vi "Grab with Bayer Decoding -ajg.vi"() -> ()   [LabVIEW 2020]
doc: "The Grab with Bayer Decoding VI acquires images continuously and displays the decoded Bayer image as an RGB image in an image control on the front panel. \n\nIMAQ Create Bayer LUT configures the gains to apply to the color planes. Refer to the Bayer decoding documentation in the White Balancing Utility for more information about setting the appropriate gains. Initialize the LUT only once to minimize decoding time. IMAQ Bayer Color Decode decodes a monochrome image to create the RGB image. An image control displays the RGB image on the front panel. After exiting the loop, IMAQ Extract Buffer releases the last extracted buffer. IMAQ Close releases resources associated with the acquisition, and IMAQ Dispose frees the buffers used for acquisition and Bayer decoding."
panel:
  out "error out 4":errorcluster
  out "error out 3":errorcluster
  out "error out 2":errorcluster
  out "Image 2":T1(plugin-control)
  out "error out":errorcluster
  in  "milliseconds to wait":u32=200
  in  "File Path":path=path "c:/temp"
  in  "Save":bool
  in  "Bayer Decoding Parameters":T2={"Bayer Pattern"=0, "Decode Method"=0, "Red Gain"=1.0, "Blue Gain"=1.0, "Green Gain"=1.0} {"Green Gain" min=0.0 max=3.99 step=0.01; "Blue Gain" min=0.0 max=3.99 step=0.01; "Red Gain" min=0.0 max=3.99 step=0.01; "Decode Method" items=["Bilinear", "VNG"]; "Bayer Pattern" items=["GBGB::RGRG", "GRGR::BGBG", "BGBG::GRGR", "RGRG::GBGB"]}
  out "Image":T1(plugin-control)
  out "Buffer Number":u32
  in  "Interface Name":string="img0"
  in  "Stop":bool
  # "Overview: Demonstrates how to perform a continuous acquisition and decode Bayer images to a color image.\nRequirements: Vision Acquisition Software, IMAQ frame grabber.\nInstructions: \n1. Select the IMAQ frame grabber Interface Name.\n2. Run the VI.\n3. If the camera file associated with the Interface Name does not already have Bayer settings defined, you can adjust the gains and Bayer Pattern. Otherwise, you can only adjust the gains."
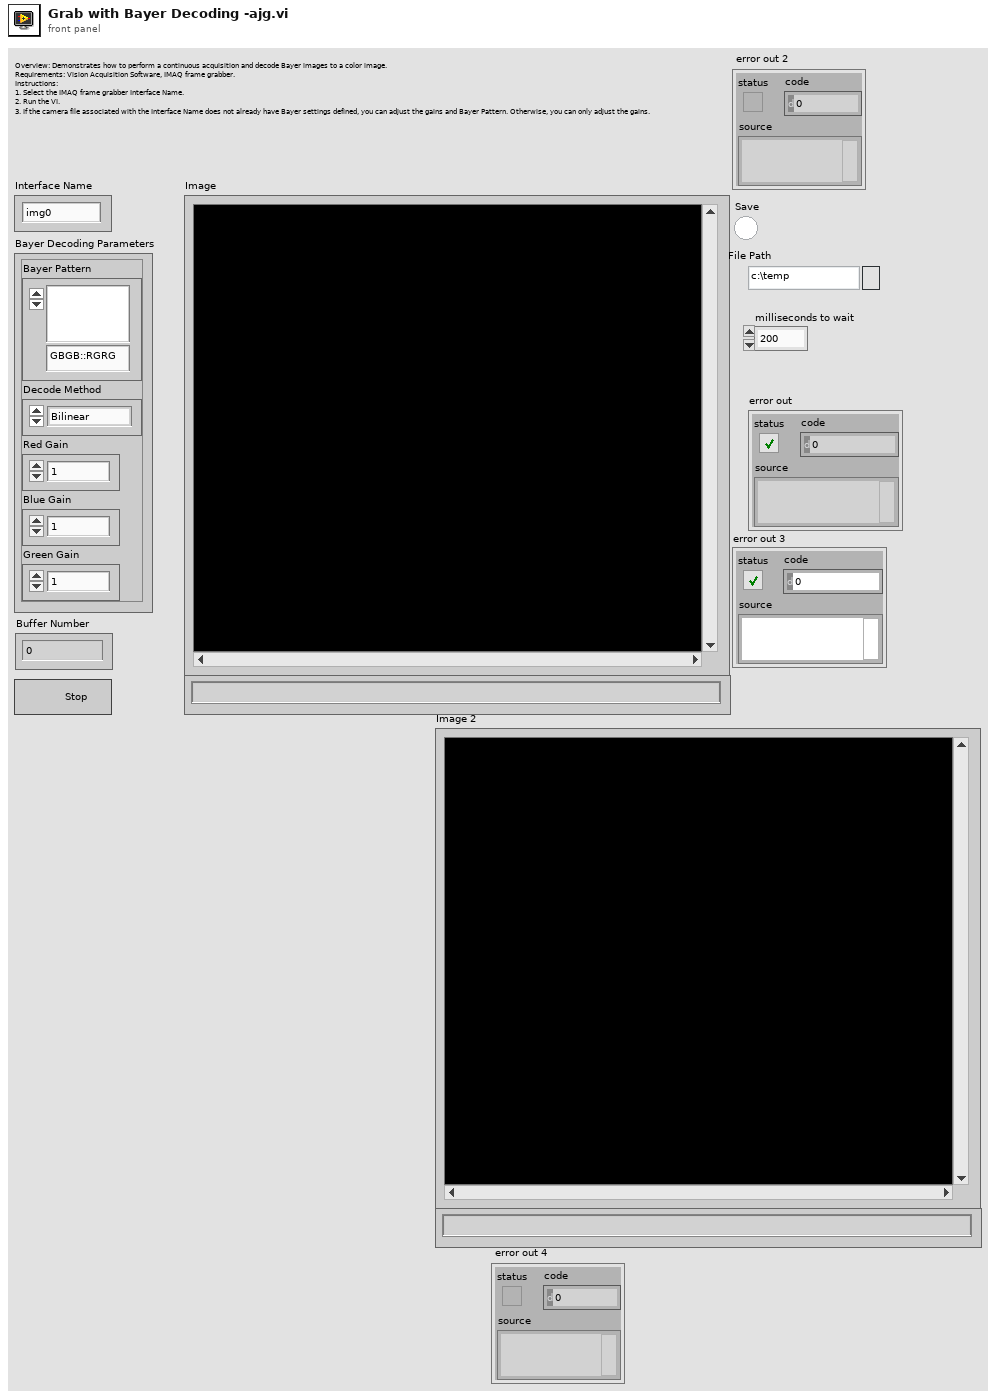
[diagram p1: front panel]
types:
  T1 = typedef "IMAQ Image.ctl" = refnum<image>
  T2 = cluster{"Bayer Pattern":i32, "Decode Method":i32, "Red Gain":dbl, "Blue Gain":dbl, "Green Gain":dbl}
  T3 = typedef "Image Type" = u32
  T4 = enum8{"Enabled", "Disabled", "Disabled and Grayed Out"}
  T5 = cluster{"Bayer Pattern":i32, "Decode Method":i32, "Bayer Red Gain":dbl, "Bayer Green Gain":dbl, "Bayer Blue Gain":dbl}
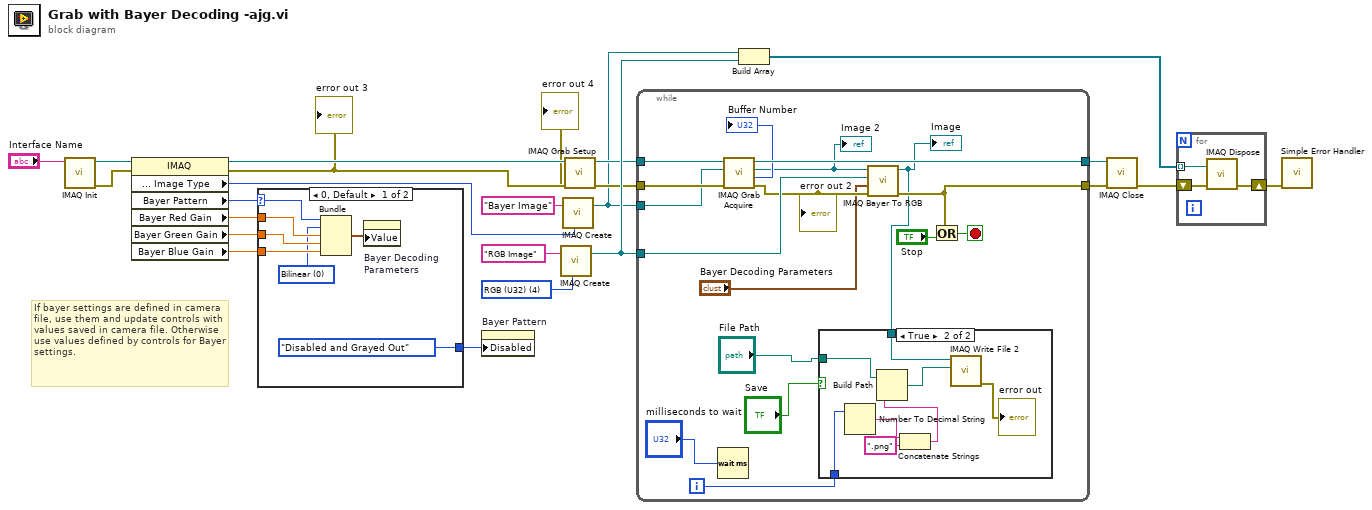
[diagram p0: block diagram]
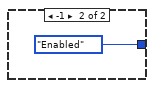
[diagram p2: hidden frame]
diagram:
  w18 = T3 4 items=["Grayscale (U8)", "Grayscale (I16)", "Grayscale (SGL)", "Complex (CSG)", "RGB (U32)", "HSL (U32)", "RGB (U64)", "Grayscale (U16)"] ("Image Type")
  # "If bayer settings are defined in camera file, use them and update controls with values saved in camera file. Otherwise use values defined by controls for Bayer settings."
  n1 = call <vilib>:"IMAQ Init.vi"("Interface Name"="Interface Name") -> ("error out"=w11:errorcluster, "IMAQ Session Out"=w12:refnum<k11>)  [unwired: 1 in, 8 out]
  n2 = property class="IMAQ"(reference=w12, error in=w11) -> (reference out=w10:refnum<k11>, error out=w9:errorcluster, "Image Parameters : Image Type"=w5:u32, "Bayer Pattern"=w16:i32, "Bayer Red Gain"=w15:dbl, "Bayer Green Gain"=w14:dbl, "Bayer Blue Gain"=w13:dbl)
  "error out 3" <- w9
  n3 = case shown="0, Default" w16 {
    selector: w16 -> [w26 _]
    tunnel: w15 -> [w29 _]
    tunnel: w14 -> [w28 _]
    tunnel: w13 -> [w27 _]
    tunnel: [T4."Disabled and Grayed Out" ("Disabled") T4."Enabled" ("Disabled")] -> w4
    frame 0, Default {
      w24 = 0 items=["Bilinear", "VNG"] ("Decode Method")
      n4 = Bundle("Bayer Pattern"=w26, "Decode Method"=w24, "Bayer Red Gain"=w29, "Bayer Green Gain"=w28, "Bayer Blue Gain"=w27) -> (w25:T5)  [unwired: 1 in]
      n5 = property on="Bayer Decoding Parameters" class="Clust (strict)"("Value"=w25) -> ()  [unwired: 2 in, 2 out]
    }
    frame -1 {
    }
  }
  n6 = property on="Bayer Pattern" class="Ring (strict)"("Disabled"=w4) -> ()  [unwired: 2 in, 2 out]
  n7 = call "IMAQ Create"("Image Name"="RGB Image", "Image Type"=w18) -> ("New Image"=w17:T1)  [unwired: 2 in, 2 out]
  n8 = call "IMAQ Create"("Image Name"="Bayer Image", "Image Type"=w5) -> ("New Image"=w3:T1)  [unwired: 2 in, 2 out]
  n9 = call <vilib>:"IMAQ Grab Setup.vi"("error in (no error)"=w9, "IMAQ Session In"=w10) -> ("error out"=w8:errorcluster, "IMAQ Session Out"=w7:refnum<k11>)  [unwired: 8 in]
  "error out 4" <- w8
  n10 = while {
    tunnel: w17 -> [w41]
    tunnel: [w45] -> w2
    tunnel: w7 -> [w46]
    tunnel: w8 -> [w44]
    tunnel: [w40] -> w1
    tunnel: w3 -> [w42]
    i -> [w35]
    stop <- w47 stop-if-true
    n11 = Wait (ms)(milliseconds to wait="milliseconds to wait") -> ()  [unwired: 1 out]
    n12 = call <vilib>:"IMAQ Grab Acquire.vi"("error in (no error)"=w44, "Image In"=w42, "IMAQ Session In"=w46) -> ("error out"=w39:errorcluster, "Acquired Buffer Number"=→"Buffer Number":u32, "Image Out"=w32:T1, "IMAQ Session Out"=w45:refnum<k11>)  [unwired: 5 in]
    "Image 2" <- w32
    "error out 2" <- w39
    n13 = call "IMAQ Bayer To RGB"("error in (no error)"=w39, "Bayer Parameters"="Bayer Decoding Parameters", "Image Dst"=w41, "Image Src"=w32) -> ("error out"=w40:errorcluster, "Image Dst Out"=w33:T1)  [unwired: 6 in]
    "Image" <- w33
    n14 = case shown="True" "Save" {
      tunnel: "File Path" -> [_ w56]
      tunnel: w35 -> [_ w53]
      tunnel: w33 -> [_ w51]
      frame False {
      }
      frame True {
        n15 = Number To Decimal String(number=w53) -> (decimal integer string=w55:string)  [unwired: 1 in]
        n16 = Concatenate Strings(w55, ".png" ("string")) -> (w52:string)
        n17 = Build Path(base path=w56, name or relative path=w52) -> (appended path=w50:path)
        n18 = call-poly "IMAQ Write File 2"("File Path"=w50, "Image"=w51) -> ("error out"=→"error out":errorcluster)  [unwired: 8 in, 1 out]
      }
    }
    n19 = Or(x=w40, y="Stop") -> (x .or. y?=w47:bool)
  }
  n20 = Build Array(w3, w17) -> (w21:T1[])
  n21 = call <vilib>:"IMAQ Close.vi"("error in (no error)"=w1, "IMAQ Session In"=w2) -> ("error out"=w20:errorcluster)  [unwired: 9 out]
  n22 = for {
    tunnel: w21 -> [w59] mode=indexing
    shift-right: [w57] -> w19
    shift-left: w20 -> [w58]
    n23 = call "IMAQ Dispose"("Image"=w59, "error in (no error)"=w58) -> ("error out"=w57:errorcluster)  [unwired: 1 in, 3 out]
  }
  n24 = call <vilib>:"Simple Error Handler.vi"("error in (no error)"=w19) -> ()  [unwired: 1 in, 8 out]
